vi "AxisCutter.vi"(0 "수신":string) -> (1 "L":i32, 2 "R":i32, 3 "C":i32, 4 "Axis":string)   [LabVIEW 2013]
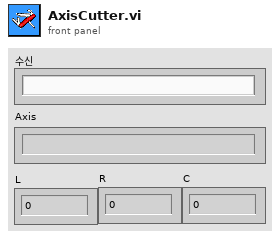
[diagram p1: front panel]
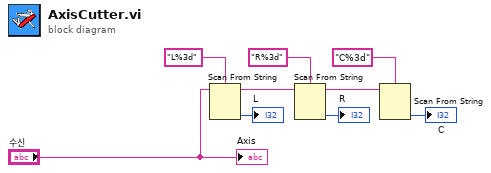
[diagram p0: block diagram]
diagram:
  n1 = Scan From String(format string="L%3d" ("포맷 문자열"), input string="수신") -> (remaining string=w6:string, output 1=→"L":i32)  [unwired: 3 in, 2 out]
  n2 = Scan From String(format string="R%3d" ("포맷 문자열"), input string=w6) -> (remaining string=w4:string, output 1=→"R":i32)  [unwired: 3 in, 2 out]
  n3 = Scan From String(format string="C%3d" ("포맷 문자열"), input string=w4) -> (output 1=→"C":i32)  [unwired: 3 in, 3 out]
  "Axis" <- "수신"
